vi "find missing channels.vi"(9 "known channels":refnum<class "TBM channel.lvclass">[](array[class]), 10 "current classification":T4, 11 "known mappings":T1[](array[typedef])) -> (3 "missing channels":refnum<class "TBM channel.lvclass">[](array[class]))   [LabVIEW 2013, in "engine configuration.lvclass"]
uses:
  engine configuration.lvclass
  <vilib>/NI/Tag Bus Module Framework/channel/TBM channel.lvclass
  <vilib>/NI/Tag Bus Module Framework/channel/channel classification.ctl
  <vilib>/NI/Tag Bus/table/mapping specification.ctl
  <vilib>/NI/Tag Bus/tag/Data Type.ctl
  <vilib>/NI/Tag Bus/table/mapping.ctl
  <vilib>/NI/Tag Bus Module Framework/channel/TBM channel.lvclass/TBM channel.ctl
  <vilib>/NI/Tag Bus/tag/tag descriptor.lvclass/tag descriptor.ctl
  <vilib>/NI/Tag Bus/tag/read tag name.vi
  <vilib>/NI/Tag Bus/tag/tag descriptor.lvclass
  <vilib>/NI/Tag Bus/table/data table.lvlib
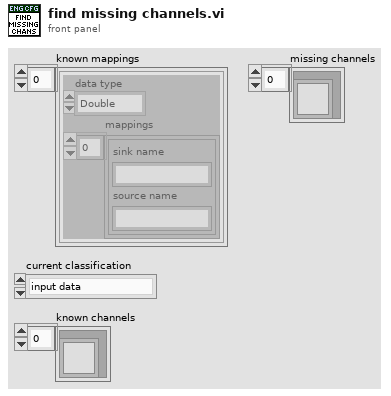
[diagram p1: front panel]
types:
  T1 = typedef "tag bus.lvlib/data table.lvlib/mapping specification.ctl" = cluster{"data type":T2, "mappings":T3[]}
  T2 = typedef "tag bus.lvlib/tag descriptor.lvclass/Data Type.ctl" = enum16{"Double", "Single", "I64", "I32", "I16", "I8", "U64", "U32", "U16", "U8", "Boolean", "String", "Array of Double", "Array of Single", "Array of I64", "Array of I32", "Array of I16", "Array of I8", "Array of U64", "Array of U32", "Array of U16", "Array of U8", "Array of Boolean", "Array of String"}
  T3 = typedef "tag bus.lvlib/data table.lvlib/mapping.ctl" = cluster{"sink name":string, "source name":string}
  T4 = typedef "TBM channel.lvclass/channel classification.ctl" = enum16{"input data", "output data", "processing parameter", "processing result"}
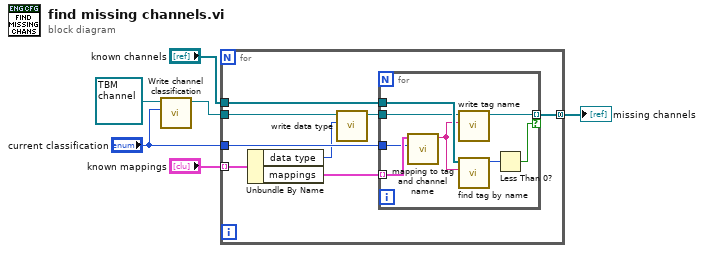
[diagram p0: block diagram]
diagram:
  n1 = call <vilib>:"Write channel classification.vi"("channel classification"="current classification", "channel in"=refnum<class "TBM channel.lvclass"> refnum) -> ("channel out"=w5:refnum<class "TBM channel.lvclass">)  [unwired: 8 in, 1 out]
  n2 = for {
    tunnel: "known channels" -> [w14]
    tunnel: "known mappings" -> [w13] mode=indexing
    tunnel: "current classification" -> [w11]
    tunnel: w5 -> [w10]
    tunnel: [w7] -> w6 mode=concatenating
    n3 = Unbundle By Name(w13) -> ("data type"=w9:T2, "mappings"=w12:T3[])
    n4 = call <vilib>:"write data type.vi"("data type"=w9, "system tag in"=w10) -> ("system tag out"=w8:refnum<class "TBM channel.lvclass">)  [unwired: 8 in, 1 out]
    n5 = for {
      tunnel: w14 -> [w22]
      tunnel: w12 -> [w21] mode=indexing
      tunnel: w11 -> [w20]
      tunnel: w8 -> [w19]
      tunnel: [w18] -> w7 mode=indexing if=w15
      n6 = call "mapping to tag and channel name.vi"("channel classification"=w20, "mapping"=w21) -> ("channel"=w17:string)  [unwired: 8 in, 1 out]
      n7 = call <vilib>:"write tag name.vi"("name"=w17, "system tag in"=w19) -> ("system tag out"=w18:refnum<class "TBM channel.lvclass">)  [unwired: 8 in, 1 out]
      n8 = call <vilib>:"find tag by name.vi"("name"=w17, "tags in"=w22) -> ("index"=w16:i32)  [unwired: 9 in]
      n9 = Less Than 0?(x=w16) -> (x < 0?=w15:bool)
    }
  }
  "missing channels" <- w6
